vi "Set Microgrid ID.vi"(8 "error in":errorcluster, 11 "IED in":refnum<class "IED.lvclass">) -> (0 "error out":errorcluster, 3 "IED out":refnum<class "IED.lvclass">)   [LabVIEW 2018, in "IED Actor.lvlib" / "IED.lvclass"]
doc: "Publishes a DDS message to set the MicrogridID of an IED specified by DeviceID."
uses:
  IED.lvclass
  C:/Users/Administrator/Desktop/2018LabVIEW EMS/EMS Generic Actor/EMS Generic/EMS Generic.lvclass
  C:/Users/Administrator/Desktop/2018LabVIEW EMS/IED Actors/Device DDS Communications Framework/Device DDS Communications/Device DDS Communications.lvclass
  Device DDS Communications Framework/Device DDS Communications/Device DDS Communications.lvclass/Device DDS Communications.ctl
  <vilib>/ORNL/CSEISMIC DDS/CSEISMIC DDS Base/Data Types/IED_setMicrogridID.ctl
  <vilib>/ORNL/CSEISMIC DDS/CSEISMIC DDS Base/Data Types/Controls/DeviceID.ctl
  <vilib>/ORNL/CSEISMIC DDS/CSEISMIC DDS Base/CSEISMIC DDS.lvclass/CSEISMIC DDS.ctl
  <vilib>/ORNL/CSEISMIC DDS/CSEISMIC DDS Base/Accessors/Read DDS Reference.vi
  <vilib>/ORNL/CSEISMIC DDS/DDS Writer/DDS Writer.lvclass
  C:/Program Files (x86)/National Instruments/LabVIEW 2018/vi.lib/ORNL/CSEISMIC DDS/CSEISMIC DDS Base/CSEISMIC DDS.lvclass
  <vilib>/ORNL/CSEISMIC DDS/CSEISMIC DDS Base/Error Handler.vi
  Device DDS Communications Framework/Device DDS Communications/Device DDS Communications.lvclass
  <vilib>/ORNL/CSEISMIC DDS/CSEISMIC DDS Base/CSEISMIC DDS.lvclass
  EMS Generic Actor/EMS Generic/EMS Generic.lvclass
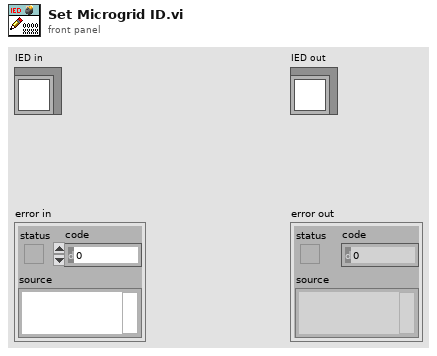
[diagram p1: front panel]
types:
  T1 = typedef "CSEISMIC DDS.lvlib/CSEISMIC DDS.lvclass/IED_setMicrogridID.ctl" = cluster{"DeviceID":T2, "MicrogridID":u8}
  T2 = typedef "CSEISMIC DDS.lvlib/CSEISMIC DDS.lvclass/DeviceID.ctl" = string
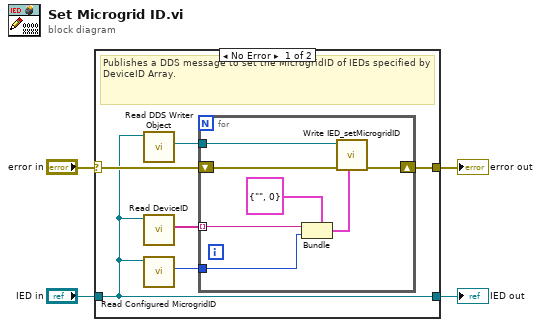
[diagram p0: block diagram]
diagram:
  n1 = case shown="No Error" "error in" {
    selector: "error in" -> [w10 w19]
    tunnel: [w9 w19] -> w3
    tunnel: [w7 w18] -> w1
    tunnel: "IED in" -> [w7 w18]
    frame No Error {
      # "Publishes a DDS message to set the MicrogridID of IEDs specified by DeviceID Array."
      n2 = call "Read DDS Writer Object.vi"("Device DDS Communications in"=w7) -> ("DDS Writer Object"=w6:refnum<class "DDS Writer.lvclass">)  [unwired: 9 in, 1 out]
      n3 = call-dynamic "Read DeviceID.vi"("Device DDS Communications in"=w7) -> ("DeviceID"=w5:T2[])  [unwired: 9 in, 1 out]
      n4 = call "Read Configured MicrogridID.vi"("EMS Generic in"=w7) -> ("Microgrid ID"=w8:u8)  [unwired: 8 in, 2 out]
      n5 = for {
        tunnel: w6 -> [w13]
        shift-right: [w14] -> w9
        shift-left: w10 -> [w15]
        tunnel: w5 -> [w11] mode=indexing
        tunnel: w8 -> [w16]
        n6 = Bundle(cluster=T1 {"DeviceID"="", "MicrogridID"=0} ("Cluster"), "DeviceID"=w11, "MicrogridID"=w16) -> (w12:T1)
        n7 = call <vilib>:"Write IED_setMicrogridID.vi"("IED_setMicrogridID"=w12, "error in"=w15, "DDS Writer in"=w13) -> ("error out"=w14:errorcluster)  [unwired: 7 in, 1 out]
      }
    }
    frame Error {
    }
  }
  "error out" <- w3
  "IED out" <- w1
